vi "PSCHN_Checking Symbols.vi"(8 "error in (no error)":errorcluster caption="错误输入（无错误）", 9 "Cards":T1[](array[typedef]), 10 "Tag":string, 11 "CfgList Tree":refnum<vi>) -> (0 "error out":errorcluster caption="错误输出", 1 "Cards Out":T1[](array[typedef]))   [LabVIEW 2016]
uses:
  Controls/PSCHN_Card Para.ctl
  Controls/PSCHN_Channel Para.ctl
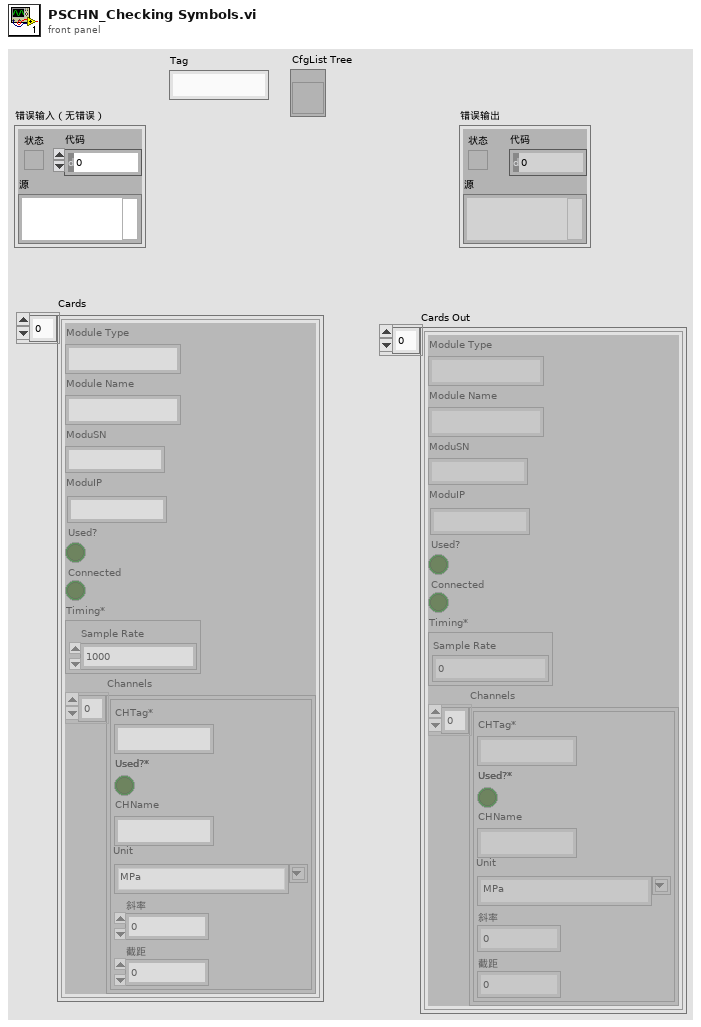
[diagram p1: front panel]
types:
  T1 = typedef "PSCHN_Card Para.ctl" = cluster{"Module Type":string, "Module Name":string, "ModuSN":string, "ModuIP":string, "Used?":bool, "Connected":bool, "Timing*":cluster{"Sample Rate":dbl}, "Channels":T2[]}
  T2 = typedef "PSCHN_Channel Para.ctl" = cluster{"CHTag*":string, "Used?*":bool, "CHName":string, "Unit":string, "斜率":dbl, "截距":dbl}
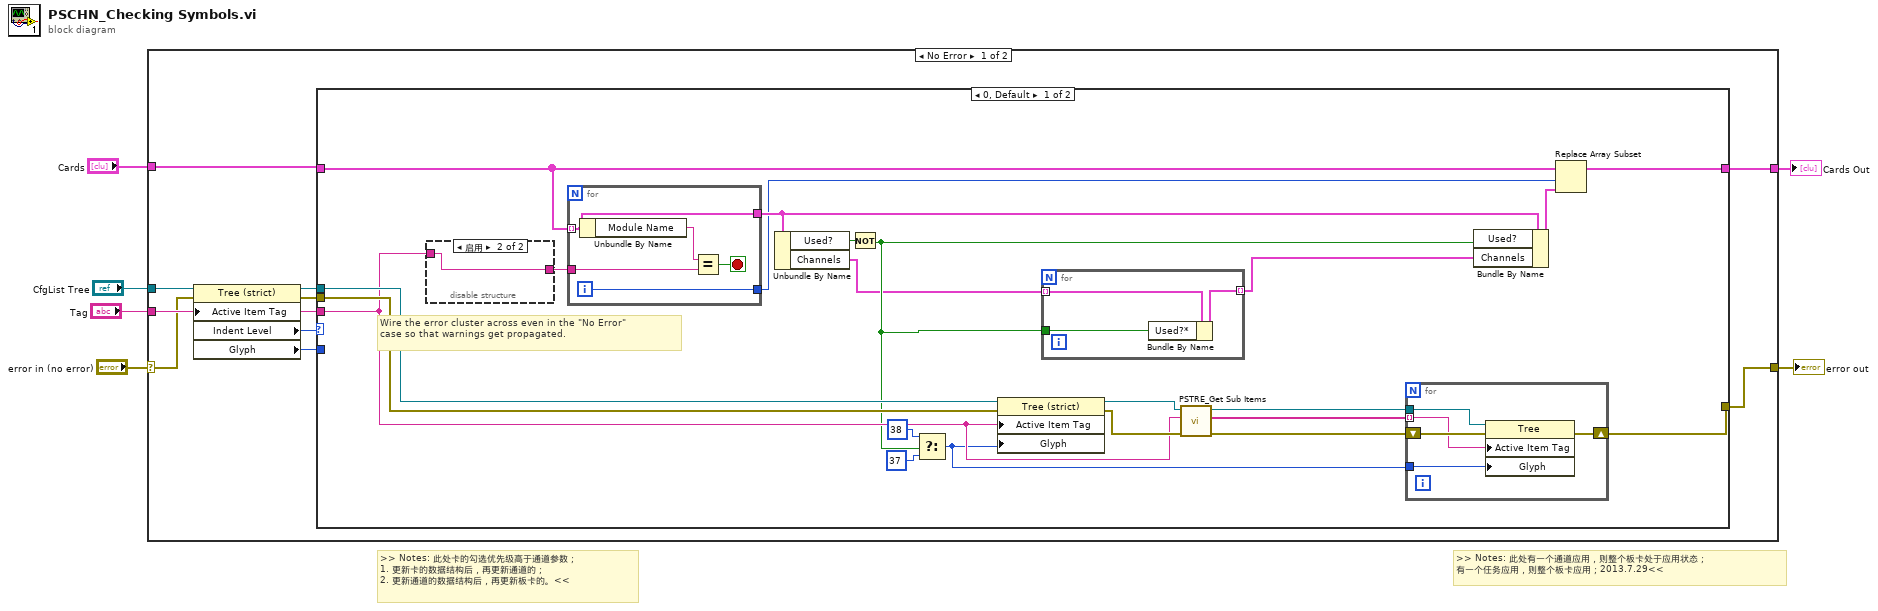
[diagram p0: block diagram]
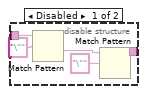
[diagram p2: hidden frame]
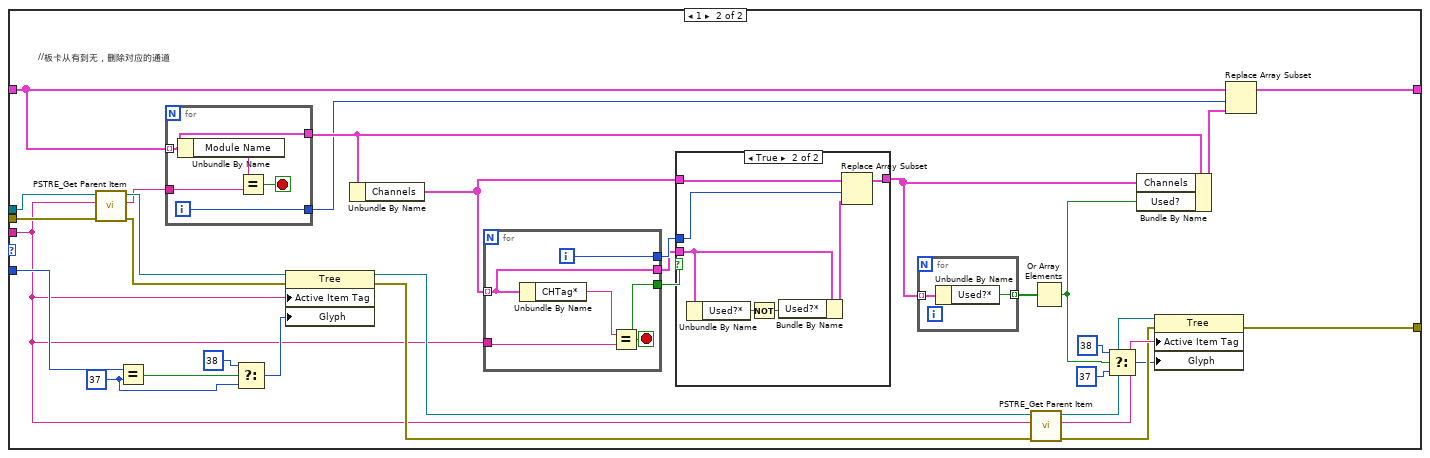
[diagram p3: hidden frame]
diagram:
  # ">> Notes: 此处有一个通道应用，则整个板卡处于应用状态；\n有一个任务应用，则整个板卡应用；2013.7.29<<"
  # ">> Notes: 此处卡的勾选优先级高于通道参数；\n1. 更新卡的数据结构后，再更新通道的；\n2. 更新通道的数据结构后，再更新板卡的。<<"
  n1 = case shown="No Error" "error in (no error)" {
    selector: "error in (no error)" -> [w12 w111]
    tunnel: [w10 w111] -> w5
    tunnel: "CfgList Tree" -> [w14 _]
    tunnel: "Tag" -> [w13 _]
    tunnel: "Cards" -> [w8 w110]
    tunnel: [w7 w110] -> w1
    frame No Error {
      # "Wire the error cluster across even in the \"No Error\"\ncase so that warnings get propagated."
      n2 = property class="Tree (strict)"(reference=w14, error in=w12, "Active Item Tag"=w13) -> (reference out=w16:refnum<vi>, error out=w11:errorcluster, "Indent Level"=w15:i32, "Glyph"=w9:i32)
      n3 = case shown="0, Default" w15 {
        tunnel: w13 -> [w25 w66]
        tunnel: w16 -> [w31 w89]
        tunnel: w11 -> [w30 w88]
        tunnel: w8 -> [w35 w86]
        tunnel: [w32 w84] -> w7
        tunnel: [w20 w71] -> w10
        tunnel: w9 -> [_ w80]
        frame 0, Default {
          n4 = disable-structure shown="启用" {
            disable-tunnel: [w43 w44] -> w38
            disable-tunnel: w25 -> [w39 w44]
            frame Disabled {
              n5 = Match Pattern(string=w39, regular expression="\"") -> (after substring=w42:string)  [unwired: 1 in, 3 out]
              n6 = Match Pattern(string=w42, regular expression="\"") -> (before substring=w43:string)  [unwired: 1 in, 3 out]
            }
            frame Enabled {
            }
          }
          n7 = for {
            tunnel: w35 -> [w54] mode=indexing
            tunnel: w38 -> [w56]
            tunnel: [w54] -> w37
            tunnel: [w53] -> w33
            i -> [w53]
            stop <- w55 stop-if-true
            n8 = Unbundle By Name(w54) -> ("Module Name"=w57:string)
            n9 = Equal?(x=w57, y=w56) -> (x = y?=w55:bool)
          }
          n10 = Unbundle By Name(w37) -> ("Used?"=w36:bool, "Channels"=w18:T2[])
          n11 = Not(x=w36) -> (.not. x?=w19:bool)
          n12 = Select(t=38 ("Active Item:Symbol Index"), s=w19, f=37 ("Active Item:Symbol Index")) -> (s? t:f=w21:i32)
          n13 = property class="Tree (strict)"(reference=w31, error in=w30, "Active Item Tag"=w25, "Glyph"=w21) -> (reference out=w27:refnum<vi>, error out=w26:errorcluster)
          n14 = for {
            tunnel: w18 -> [w45] mode=indexing
            tunnel: [w47] -> w17 mode=indexing
            tunnel: w19 -> [w46]
            n15 = Bundle By Name(cluster=w45, "Used?*"=w46) -> (w47:T2)
          }
          n16 = call <vilib>:"PSTRE_Get Sub Items.vi"("error in"=w26, "Par Tag"=w25, "TreeRef"=w27) -> ("error out"=w23:errorcluster, "Tags"=w22:string[], "TreeRef"=w24:refnum<vi>)  [unwired: 5 in, 1 out]
          n17 = for {
            tunnel: w24 -> [w52]
            tunnel: w22 -> [w49] mode=indexing
            shift-right: [w50] -> w20
            shift-left: w23 -> [w51]
            tunnel: w21 -> [w48]
            n18 = property class="Tree"(reference=w52, error in=w51, "Active Item Tag"=w49, "Glyph"=w48) -> (error out=w50:errorcluster)  [unwired: 1 out]
          }
          n19 = Bundle By Name(cluster=w37, "Used?"=w19, "Channels"=w17) -> (w34:T1)
          n20 = Replace Array Subset(array=w35, new element=w34, index=w33) -> (w32:T1[])
        }
        frame 1 {
          w78 = 37 ("y")
          # "//板卡从有到无，删除对应的通道"
          n21 = call <vilib>:"PSTRE_Get Parent Item.vi"("error in"=w88, "Tag"=w66, "TreeRef"=w89) -> ("error out"=w82:errorcluster, "Par Tag"=w58:string, "TreeRef"=w81:refnum<vi>)  [unwired: 5 in, 1 out]
          n22 = Equal?(x=w80, y=w78) -> (x = y?=w67:bool)
          n23 = for {
            tunnel: w86 -> [w106] mode=indexing
            tunnel: w58 -> [w108]
            tunnel: [w106] -> w87
            tunnel: [w105] -> w83
            i -> [w105]
            stop <- w107 stop-if-true
            n24 = Unbundle By Name(w106) -> ("Module Name"=w109:string)
            n25 = Equal?(x=w109, y=w108) -> (x = y?=w107:bool)
          }
          n26 = Select(t=38 ("y"), s=w67, f=w78) -> (s? t:f=w77:i32)
          n27 = property class="Tree"(reference=w81, error in=w82, "Active Item Tag"=w66, "Glyph"=w77) -> (reference out=w75:refnum<vi>, error out=w76:errorcluster)
          n28 = Unbundle By Name(w87) -> ("Channels"=w61:T2[])
          n29 = for {
            tunnel: w61 -> [w100] mode=indexing
            tunnel: w66 -> [w102]
            tunnel: [w104] -> w64
            tunnel: [w101] -> w65
            tunnel: [w100] -> w63
            i -> [w104]
            stop <- w101 stop-if-true
            n30 = Unbundle By Name(w100) -> ("CHTag*"=w103:string)
            n31 = Equal?(x=w103, y=w102) -> (x = y?=w101:bool)
          }
          n32 = case shown="True" w65 {
            tunnel: w64 -> [_ w95]
            tunnel: w61 -> [w92 w96]
            tunnel: [w92 w93] -> w60
            tunnel: w63 -> [_ w97]
            frame False {
            }
            frame True {
              n33 = Unbundle By Name(w97) -> ("Used?*"=w99:bool)
              n34 = Not(x=w99) -> (.not. x?=w98:bool)
              n35 = Bundle By Name(cluster=w97, "Used?*"=w98) -> (w94:T2)
              n36 = Replace Array Subset(array=w96, new element=w94, index=w95) -> (w93:T2[])
            }
          }
          n37 = for {
            tunnel: w60 -> [w91] mode=indexing
            tunnel: [w90] -> w62 mode=indexing
            n38 = Unbundle By Name(w91) -> ("Used?*"=w90:bool)
          }
          n39 = call <vilib>:"PSTRE_Get Parent Item.vi"("error in"=w76, "Tag"=w66, "TreeRef"=w75) -> ("error out"=w72:errorcluster, "Par Tag"=w74:string, "TreeRef"=w73:refnum<vi>)  [unwired: 5 in, 1 out]
          n40 = Or Array Elements(Boolean array=w62) -> (logical OR=w59:bool)
          n41 = Select(t=38 ("Active Item:Symbol Index"), s=w59, f=37 ("Active Item:Symbol Index")) -> (s? t:f=w68:i32)
          n42 = Bundle By Name(cluster=w87, "Channels"=w60, "Used?"=w59) -> (w85:T1)
          n43 = property class="Tree"(reference=w73, error in=w72, "Active Item Tag"=w74, "Glyph"=w68) -> (error out=w71:errorcluster)  [unwired: 1 out]
          n44 = Replace Array Subset(array=w86, new element=w85, index=w83) -> (w84:T1[])
        }
      }
    }
    frame Error {
    }
  }
  "error out" <- w5
  "Cards Out" <- w1
